vi "Add Status Channels.vi"(8 "error in (no error)":errorcluster, 11 "SLSC Switch Custom Device Ref in":T1 format="%.0x") -> (0 "error out":errorcluster, 3 "SLSC Switch Custom Device Ref out":T1 format="%.0x")   [LabVIEW 2017, in "SLSC Switch Scripting.lvlib"]
uses:
  SLSC Switch Scripting.lvlib
  <vilib>/NI Veristand/Custom Device API/Custom Device Item Ref.ctl
  <vilib>/NI Veristand/Custom Device API/Custom Device Channel.ctl
  <vilib>/NI Veristand/Custom Device API/Custom Device Channel Type.ctl
  SLSC Scripting Constants.vi
  <vilib>/NI Veristand/Custom Device API/Custom Device API.lvlib
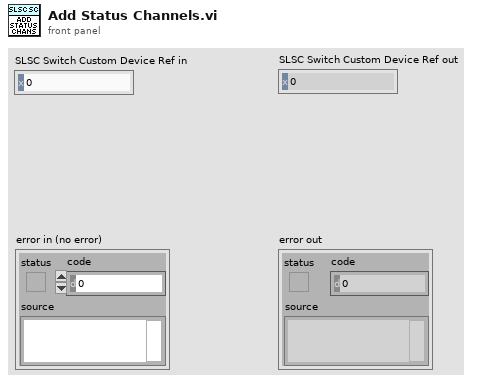
[diagram p1: front panel]
types:
  T1 = typedef "Custom Device API.lvlib/Custom Device Item Ref.ctl" = u64
  T2 = typedef "Custom Device API.lvlib/Custom Device Channel.ctl" = cluster{"Type":T3, "Units":string, "Default Value":dbl, "Faultable":bool, "Scalable":bool}
  T3 = typedef "Custom Device API.lvlib/Custom Device Channel Type.ctl" = enum16{"Input", "Output"}
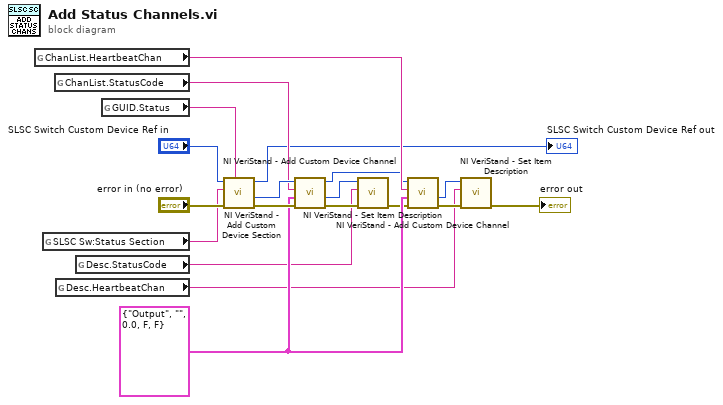
[diagram p0: block diagram]
diagram:
  w12 = T2 {"Type"=enum."Output", "Units"="", "Default Value"=0.0, "Faultable"=FALSE, "Scalable"=FALSE} ("Channel")
  n1 = global read "SLSC Scripting Constants.vi" "ChanList.HeartbeatChan"() -> (w11:string)
  n2 = global read "SLSC Scripting Constants.vi" "SLSC Sw:Status Section"() -> (w16:string)
  n3 = global read "SLSC Scripting Constants.vi" "ChanList.StatusCode"() -> (w13:string)
  n4 = global read "SLSC Scripting Constants.vi" "Desc.HeartbeatChan"() -> (w1:string)
  n5 = global read "SLSC Scripting Constants.vi" "Desc.StatusCode"() -> (w7:string)
  n6 = global read "SLSC Scripting Constants.vi" "GUID.Status"() -> (w17:string)
  n7 = call <vilib>:"NI VeriStand - Add Custom Device Section.vi"("GUID (Default Section)"=w17, "error in (no error)"="error in (no error)", "Section Name"=w16, "Parent Ref in"="SLSC Switch Custom Device Ref in") -> ("error out"=w15:errorcluster, "Section Ptr"=w14:T1, "Parent Ref out"=→"SLSC Switch Custom Device Ref out":T1)  [unwired: 4 in, 1 out]
  n8 = call <vilib>:"NI VeriStand - Add Custom Device Channel.vi"("error in (no error)"=w15, "Channel"=w12, "Channel Name"=w13, "Parent Ref in"=w14) -> ("error out"=w9:errorcluster, "Channel Ref"=w8:T1, "Parent Ref out"=w5:T1)  [unwired: 4 in, 1 out]
  n9 = call <vilib>:"NI VeriStand - Set Item Description.vi"("error in (no error)"=w9, "Description"=w7, "Item Ref in"=w8) -> ("error out"=w6:errorcluster)  [unwired: 6 in, 2 out]
  n10 = call <vilib>:"NI VeriStand - Add Custom Device Channel.vi"("error in (no error)"=w6, "Channel"=w12, "Channel Name"=w11, "Parent Ref in"=w5) -> ("error out"=w4:errorcluster, "Channel Ref"=w3:T1)  [unwired: 4 in, 2 out]
  n11 = call <vilib>:"NI VeriStand - Set Item Description.vi"("error in (no error)"=w4, "Description"=w1, "Item Ref in"=w3) -> ("error out"=→"error out":errorcluster)  [unwired: 6 in, 2 out]
